vi "Auth Request URL.vi"(10 "Client":refnum<class "Client.lvclass">, 11 "Request in":refnum<class "Request.lvclass">) -> (3 "Request URL":string)   [LabVIEW 2020, in "OAuth2.lvlib" / "Request.lvclass"]
uses:
  Request.lvclass
  Client/Client.lvclass
  Request.lvclass/Request.ctl
  OAuth2.lvlib
  HTTP Utils/HTTP Utils.lvlib
  <vilib>/IlluminatedG/lv-stream/URI/URI.lvclass
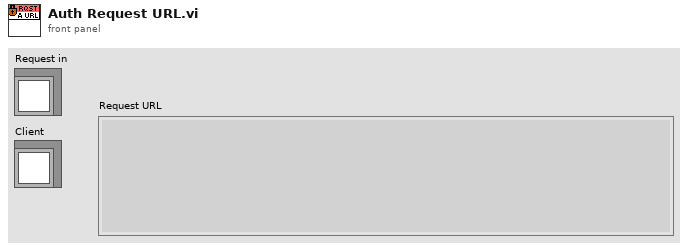
[diagram p1: front panel]
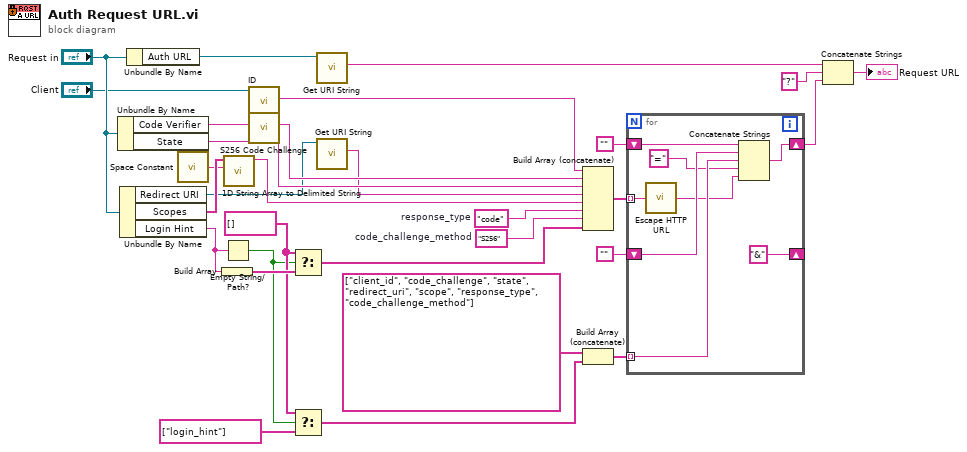
[diagram p0: block diagram]
diagram:
  w22 = "S256"  # code_challenge_method
  w23 = "code"  # response_type
  w26 = string[] []
  n1 = Unbundle By Name("Request in") -> ("Code Verifier"=w8:string, "State"=w7:string)
  n2 = Unbundle By Name("Request in") -> ("Redirect URI"=w4:refnum<class "URI.lvclass">, "Scopes"=w17:string[], "Login Hint"=w28:string)
  n3 = Unbundle By Name("Request in") -> ("Auth URL"=w6:refnum<class "URI.lvclass">)
  n4 = call <vilib>:"Space Constant.vi"() -> ("String"=w16:string)
  n5 = Build Array(w28) -> (w27:string[])
  n6 = Empty String/Path?(string/path=w28) -> (empty?=w24:bool)
  n7 = call <vilib>:"1D String Array to Delimited String.vi"("delimiter"=w16, "string array"=w17) -> ("delimited string"=w15:string)  [unwired: 9 in]
  n8 = call "ID.vi"("Client in"="Client") -> ("Client ID"=w1:string)  [unwired: 10 in]
  n9 = call "S256 Code Challenge.vi"("Code Verifier"=w8) -> ("Code Challenge"=w18:string)  [unwired: 10 in]
  n10 = Select(t=w26, s=w24, f=w27) -> (s? t:f=w20:string[])
  n11 = Select(t=w26, s=w24, f=string[] ["login_hint"]) -> (s? t:f=w13:string[])
  n12 = call <vilib>:"Get URI String.vi"("URI in"=w6) -> ("URI String"=w5:string)  [unwired: 8 in, 2 out]
  n13 = call <vilib>:"Get URI String.vi"("URI in"=w4) -> ("URI String"=w3:string)  [unwired: 8 in, 2 out]
  n14 = Build Array (concatenate)(w1, w18, w7, w3, w15, w23, w22, w20) -> (w19:string[])
  n15 = Build Array (concatenate)(string[] ["client_id", "code_challenge", "state", "redirect_uri", "scope", "response_type", "code_challenge_method"], w13) -> (w12:string[])
  n16 = for {
    tunnel: w19 -> [w38] mode=indexing
    tunnel: w12 -> [w34] mode=indexing
    shift-right: ["&"] -> _
    shift-left: "" -> [w35]
    shift-right: [w31] -> w9
    shift-left: "" -> [w36]
    n17 = call "Escape HTTP URL.vi"("unescaped string in"=w38) -> ("escaped string out"=w32:string)
    n18 = Concatenate Strings(w36, w35, w34, "=" ("string"), w32) -> (w31:string)
  }
  n19 = Concatenate Strings(w5, "?" ("string"), w9) -> (→"Request URL":string)
